vi "Get All CTRL.vi"(8 "error in (no error)":errorcluster, 11 "This VI":refnum<vi>) -> (0 "error out":errorcluster, 3 "CTRL REF":refnum<vi>[](array[refnum]))   [LabVIEW 2020]
uses:
  PCT FGV CMD.ctl
panel:
  out "Control Names":string[](array[string])
  out "Array":string[](array[string])
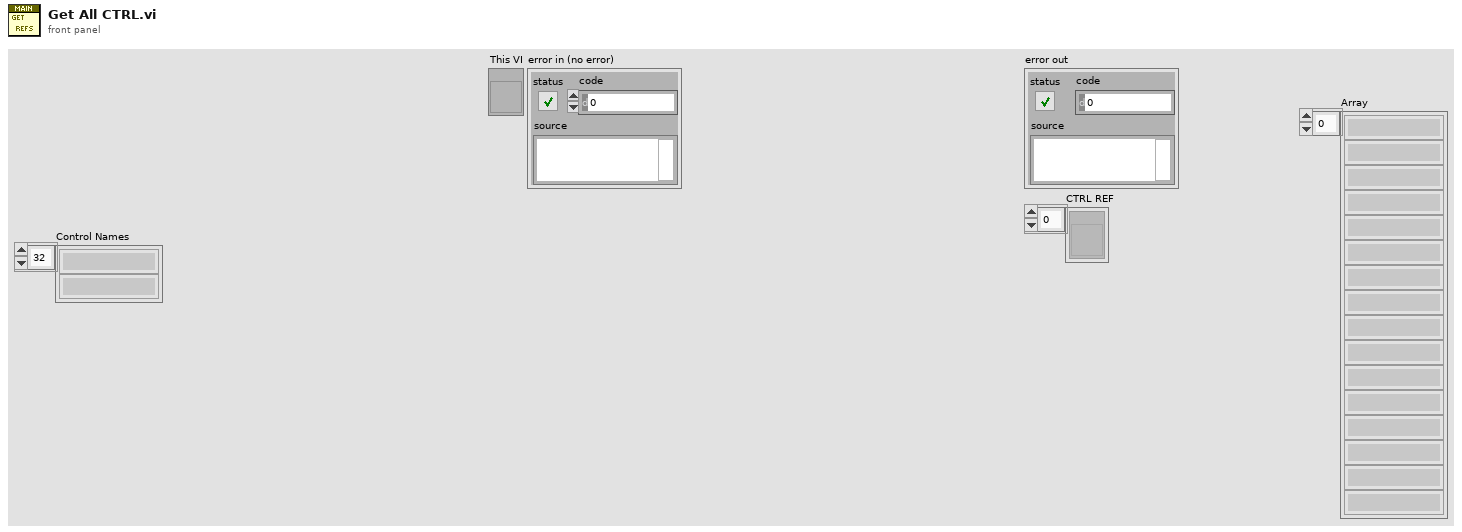
[diagram p1: front panel]
types:
  T1 = typedef "PCT FGV CMD.ctl" = enum16{"INIT", "GET", "SET"}
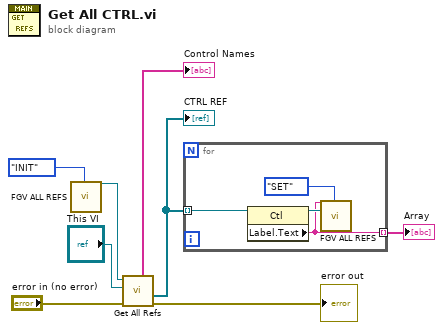
[diagram p0: block diagram]
diagram:
  n1 = call "FGV ALL REFS.vi"("CMD"=PCT_FGV_CMD."INIT") -> ("Ctl Refnum out"=w4:refnum<vi>)  [unwired: 26 in]
  n2 = call "Get All Refs.vi"("error in (no error)"="error in (no error)", "This VI"="This VI", "Control in"=w4) -> ("error out"=→"error out":errorcluster, "Controls[]"=w3:refnum<vi>[], "Label Array"=→"Control Names":string[])  [unwired: 6 in]
  "CTRL REF" <- w3
  n3 = for {
    tunnel: w3 -> [w12] mode=indexing
    tunnel: [w9] -> w7 mode=indexing
    n4 = property class="Ctl"(reference=w12) -> (reference out=w11:refnum<vi>, "Label.Text"=w9:string)  [unwired: 1 in, 1 out]
    n5 = call "FGV ALL REFS.vi"("name"=w9, "Ctl Refnum in"=w11, "CMD"=PCT_FGV_CMD."SET") -> ()  [unwired: 24 in, 1 out]
  }
  "Array" <- w7
